vi "GetCellStrColor.vi"(7 "Color":u32, 8 "error in (no error)":errorcluster, 10 "Hdr Name":T1, 11 "Thermocouple in":refnum<class "Thermocouple.lvclass">) -> (0 "error out":errorcluster, 1 "Cell String":string, 2 "Cell Color":u32, 3 "Thermocouple out":refnum<class "Thermocouple.lvclass">)   [LabVIEW 2018, in "Measurement Channels.lvlib" / "Thermocouple.lvclass"]
uses:
  Thermocouple.lvclass
  Common/Controls/HeaderNames.ctl
  SubVIs Table/Custom Ctls Table/ge_ColType.ctl
  Thermocouple.lvclass/Thermocouple.ctl
  Class Channel/Channel.lvclass
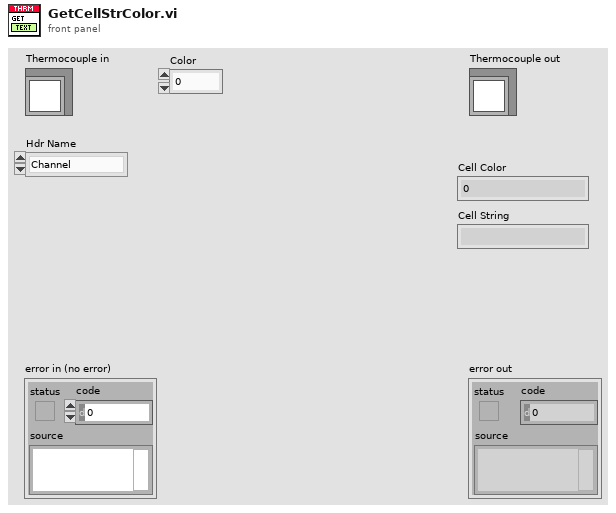
[diagram p1: front panel]
types:
  T1 = typedef "HeaderNames.ctl" = enum16{"Channel", "Device", "Spacer", "Description", "MB", "Range", "Terminal", "Coupling", "Thresh (V)", "Pulse/Rev", "Slope", "Min EU", "Min RPM", "mV/EU", "Iex", "Temp Units", "Type", "CJC Src", "CJC Val", "Ro", "Wire Cfg", "Strain Mode", "Vex", "Bridge Type", "GF", "Gauge Res", "Poisson", "Lead Res", "Init Strain", "GAF", "Scale", "Offset", "Unit (EU)", "dB?", "dB Ref", "Cal Mag", "Cal Units", "Max Temp", "Min Temp", "Max Strain", "Min Strain"}
  T2 = typedef "ge_ColType.ctl" = enum16{"Volts", "Amps", "Ohms", "TermCfg", "WireCfg", "Coup", "Slope", "Iex", "CalUnits", "ThrmUnits", "ThrmType", "CJCSrc", "BrdgType", "Strn Mode", "RTDType"}
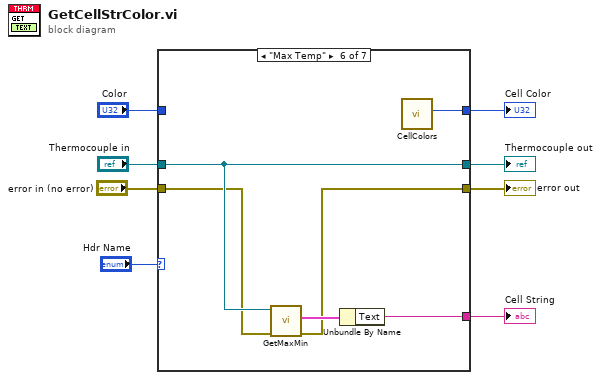
[diagram p0: block diagram]
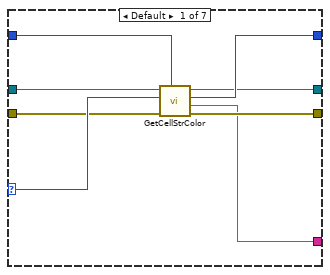
[diagram p2: hidden frame]
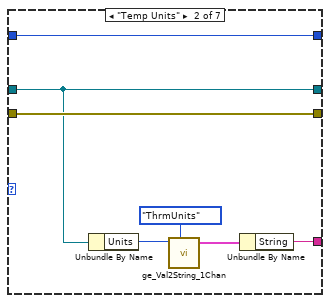
[diagram p3: hidden frame]
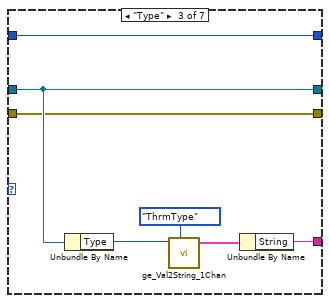
[diagram p4: hidden frame]
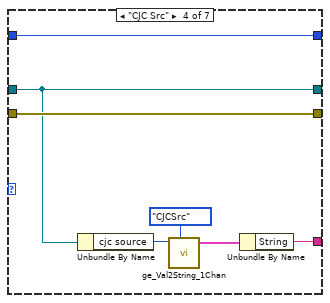
[diagram p5: hidden frame]
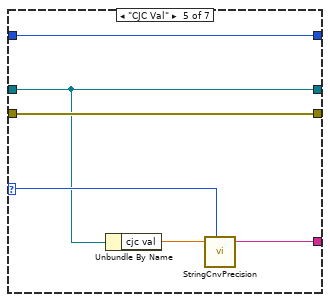
[diagram p6: hidden frame]
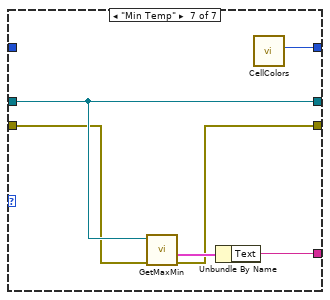
[diagram p7: hidden frame]
diagram:
  n1 = case shown="\"Max Temp\"" "Hdr Name" {
    selector: "Hdr Name" -> [w12 _ _ _ w42 _ _]
    tunnel: [w9 w22 w28 w35 w41 w47 w50] -> w1
    tunnel: "Color" -> [w13 w20 w26 w33 w39 _ _]
    tunnel: [w16 w20 w26 w33 w39 w49 w55] -> w2
    tunnel: "Thermocouple in" -> [w15 w18 w25 w31 w38 w46 w54]
    tunnel: [w14 w18 w25 w31 w38 w46 w54] -> w7
    tunnel: "error in (no error)" -> [w11 w19 w24 w32 w40 w45 w52]
    tunnel: [w10 w19 w24 w32 w40 w44 w51] -> w3
    frame Default {
      n2 = call-parent "GetCellStrColor.vi"("Color"=w13, "error in (no error)"=w11, "Hdr Name"=w12, "Channel in"=w15) -> ("error out"=w10:errorcluster, "Cell String"=w9:string, "Cell Color"=w16:u32, "Channel out"=w14:refnum<class "Thermocouple.lvclass">)  [unwired: 4 in]
    }
    frame "Temp Units" {
      n3 = Unbundle By Name(w18) -> ("Units"=w21:u16)
      n4 = call "ge_Val2String_1Chan.vi"("Value"=w21, "ColType"=ge_ColType."ThrmUnits") -> ("String and Val"=w23:cluster{"String":string, "Value":u16})  [unwired: 5 in]
      n5 = Unbundle By Name(w23) -> ("String"=w22:string)
    }
    frame "Type" {
      n6 = Unbundle By Name(w25) -> ("Type"=w27:u16)
      n7 = call "ge_Val2String_1Chan.vi"("Value"=w27, "ColType"=ge_ColType."ThrmType") -> ("String and Val"=w29:cluster{"String":string, "Value":u16})  [unwired: 5 in]
      n8 = Unbundle By Name(w29) -> ("String"=w28:string)
    }
    frame "CJC Src" {
      n9 = Unbundle By Name(w31) -> ("cjc source"=w34:u16)
      n10 = call "ge_Val2String_1Chan.vi"("Value"=w34, "ColType"=ge_ColType."CJCSrc") -> ("String and Val"=w36:cluster{"String":string, "Value":u16})  [unwired: 5 in]
      n11 = Unbundle By Name(w36) -> ("String"=w35:string)
    }
    frame "CJC Val" {
      n12 = Unbundle By Name(w38) -> ("cjc val"=w43:dbl)
      n13 = call "StringCnvPrecision.vi"("Number"=w43, "Header"=w42) -> ("Float String"=w41:string)  [unwired: 5 in]
    }
    frame "Max Temp" {
      n14 = call-dynamic "GetMaxMin.vi"("error in (no error)"=w45, "Thermocouple in"=w46) -> ("error out"=w44:errorcluster, "Max"=w48:cluster{"Value":dbl, "Text":string})  [unwired: 6 in, 2 out]
      n15 = Unbundle By Name(w48) -> ("Text"=w47:string)
      n16 = call "CellColors.vi"() -> ("Disabled"=w49:u32)  [unwired: 8 in, 3 out]
    }
    frame "Min Temp" {
      n17 = call-dynamic "GetMaxMin.vi"("error in (no error)"=w52, "Thermocouple in"=w54) -> ("error out"=w51:errorcluster, "Min"=w53:cluster{"Value":dbl, "Text":string})  [unwired: 6 in, 2 out]
      n18 = Unbundle By Name(w53) -> ("Text"=w50:string)
      n19 = call "CellColors.vi"() -> ("Disabled"=w55:u32)  [unwired: 8 in, 3 out]
    }
  }
  "error out" <- w3
  "Thermocouple out" <- w7
  "Cell String" <- w1
  "Cell Color" <- w2
